vi "String to SGL.vi"(8 "error in":errorcluster, 11 "Integer String":string) -> (0 "error out":errorcluster, 3 "SGL":sgl)   [LabVIEW 2020, in "CANopen.lvlib"]
doc: "Converts the string representation of a number in a specified base to an equivalent 32-bit signed integer."
uses:
  CANopen.lvlib
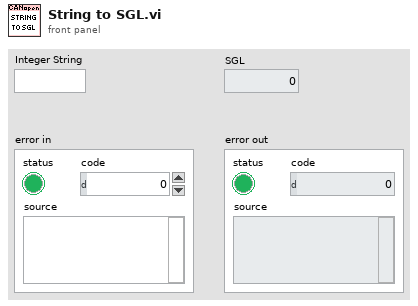
[diagram p1: front panel]
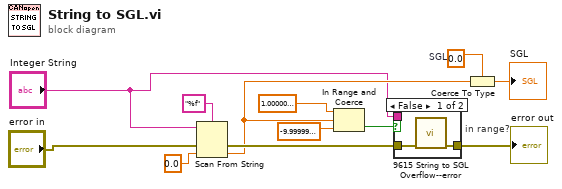
[diagram p0: block diagram]
diagram:
  w11 = sgl 0.0  # SGL
  n1 = Scan From String(format string="%f", input string="Integer String", error in="error in", default 1=0.0) -> (error out=w12:errorcluster, output 1=w5:dbl)  [unwired: 1 in, 2 out]
  n2 = In Range and Coerce(upper limit=sgl 1e+32, x=w5, lower limit=sgl -1e+37) -> (In Range?=w8:bool)  [unwired: 1 out]
  n3 = case "in range?" shown="False" w8 {
    tunnel: w12 -> [w14 w15]
    tunnel: [w13 w15] -> w4
    tunnel: "Integer String" -> [_ _]
    frame False {
      n4 = call "9615 String to SGL Overflow--error.vi"("error in"=w14) -> ("error out"=w13:errorcluster)  [unwired: 10 in]
    }
    frame True {
    }
  }
  "error out" <- w4
  n5 = Coerce To Type(0:w5, 1:w11) -> (2:→"SGL":sgl)
